vi "Test ModbusOverMOXA API.vi"() -> ()   [LabVIEW 2017]
doc: "ModbusOverMOXA API Tester."
uses:
  ModbusOverMOXA.lvlib
panel:
  in  "Write":bool
  in  "Read":bool
  in  "Len/Data":u16=1 format="%.0x"
  in  "Register":u16 format="%.0x"
  in  "Drive":bool
  in  "Hz":dbl
  in  "engage":bool
  in  "Boolean":bool
  in  "Status":bool
  in  "Local":bool
  in  "Remote":bool
  in  "config":string="{\"MQTT\":\"{\\n  \\\"Broker\\\": {\\n    \\\"IP\\\": \\\"192.168.20.249\\\",\\n    \\\"port\\\": 1883,\\n    \\\"connTimeout\\\": 3000,\\n    \\\"writeTimeout\\\": 3000,\\n    \\\"readTimeout\\\": 3000,\\n    \\\"subTimeout\\\": 3000\\n  },\\n  \\\"Connect Flags\\\": {\\n    \\\"reserved\\\": false,\\n    \\\"clean session\\\": false,\\n    \\\"will flag\\\": true,\\n    \\\"willQOS\\\": \\\"At least once\\\",\\n    \\\"will retain\\\": true,\\n    \\\"password\\\": false,\\n    \\\"user name\\\": false\\n  },\\n  \\\"Keep Alive\\\": 5000,\\n  \\\"Client Info\\\": {\\n    \\\"ClientId\\\": \\\"INVerterDriver$$$$$\\\",\\n    \\\"Will Topic\\\": \\\"InverterDriver/Online\\\",\\n    \\\"Will Message\\\": \\\"flase\\\",\\n    \\\"User Name\\\": \\\"\\\",\\n    \\\"Password\\\": \\\"\\\"\\n  }\\n}\",\"Serializer\":\"{\\n  \\\"Plugin\\\":\\\"MOXAIP\\\",\\n  \\\"IP\\\":\\\"192.168.20.119\\\",\\n  \\\"Port\\\":4002\\n}\",\"Messages\":\"{\\n  \\\"Subscriptions\\\":\\n  {\\n    \\\"Engage\\\":\\\"Inverter/Engage\\\",\\n    \\\"Drive\\\":\\\"Inverter/Drive\\\"\\n  },\\n  \\\"Broadcasts\\\":\\n  {\\n    \\\"Status\\\":\\\"Inverter/Status\\\"\\n  }\\n}\"}"
  in  "Settings Button":bool
  in  "Run as Singleton?":bool
  in  "Show Block Diagram":bool
  in  "Refresh Modules":bool
  out "Active Modules":string[](array[string])
  in  "Stop Module":bool
  in  "Select Module":i32(ring)=-1 caption="Select Module\nTo send Request to" items=["All"=-1]
  in  "Run New Module":bool
  in  "Hide Module Panel":bool
  in  "Show Module Panel":bool
  out "Status":string
  # "This VI tests the API for the Module."
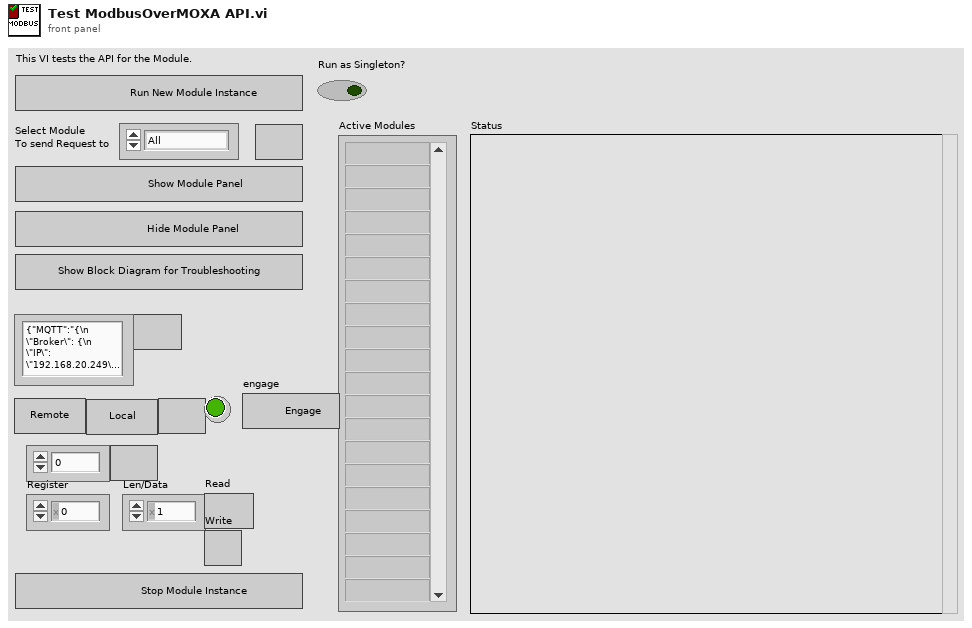
[diagram p1: front panel]
types:
  T1 = typedef "ModbusOverMOXA.lvlib/Broadcast Events--cluster.ctl" = cluster{"Module Did Init":refnum<user-event>, "Status Updated":refnum<user-event>, "Error Reported":refnum<user-event>, "Module Did Stop":refnum<user-event>, "Update Module Execution Status":refnum<user-event>}
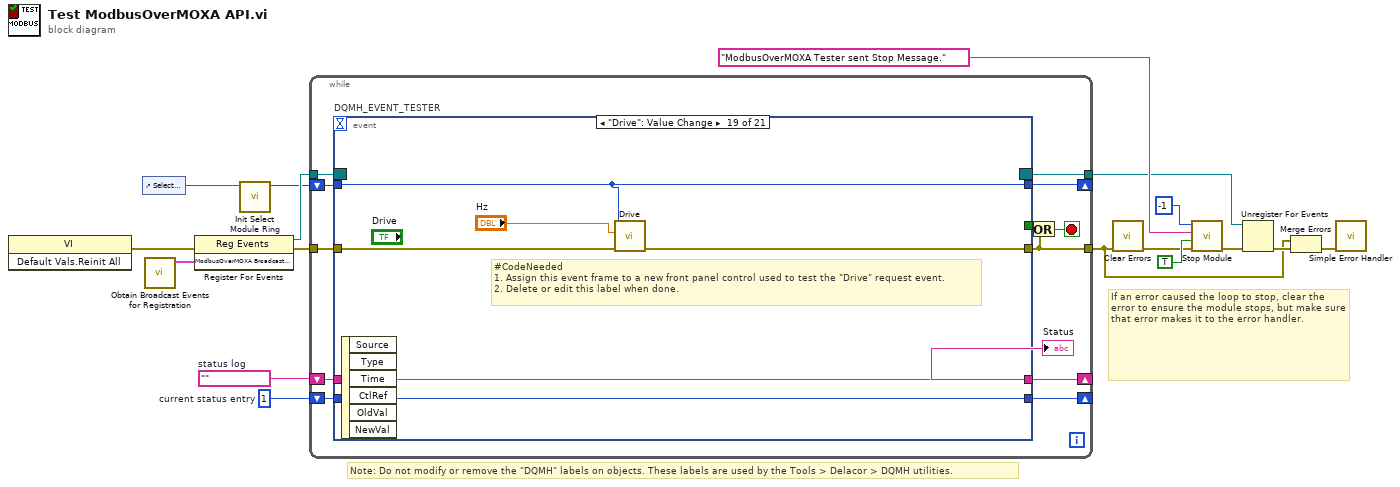
[diagram p0: block diagram]
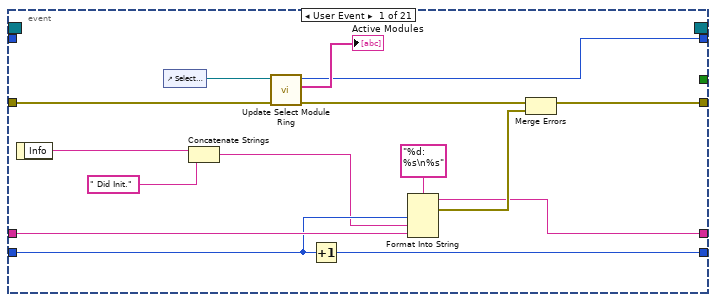
[diagram p2: hidden frame]
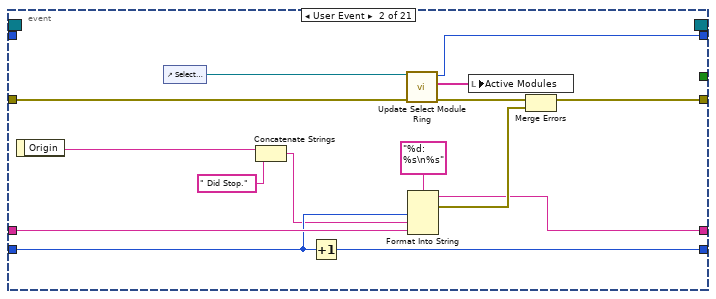
[diagram p3: hidden frame]
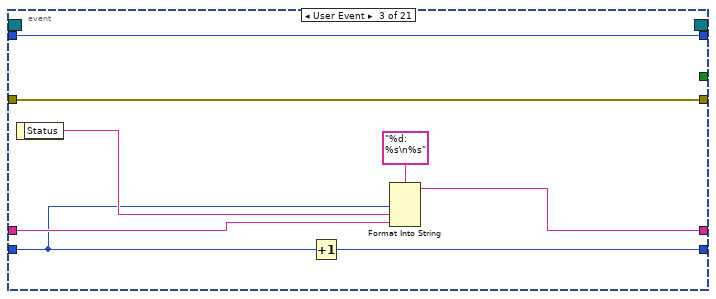
[diagram p4: hidden frame]
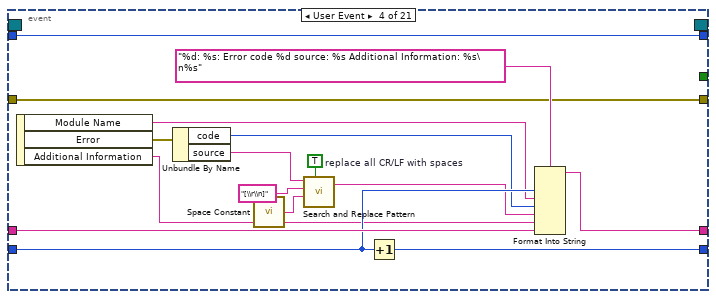
[diagram p5: hidden frame]
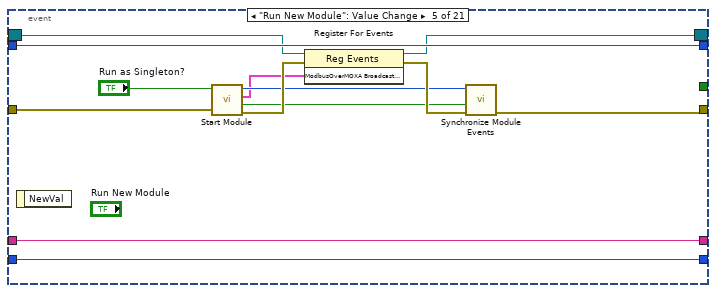
[diagram p6: hidden frame]
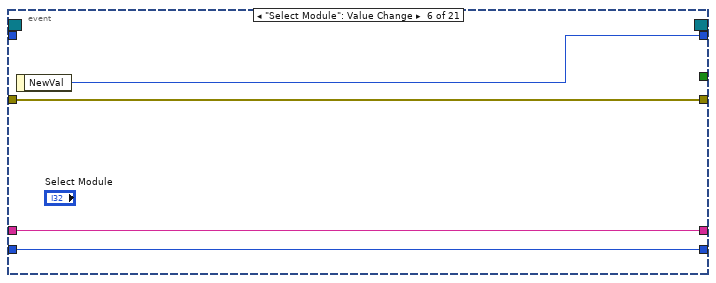
[diagram p7: hidden frame]
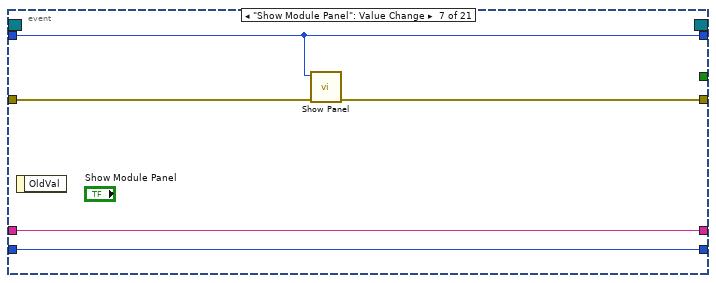
[diagram p8: hidden frame]
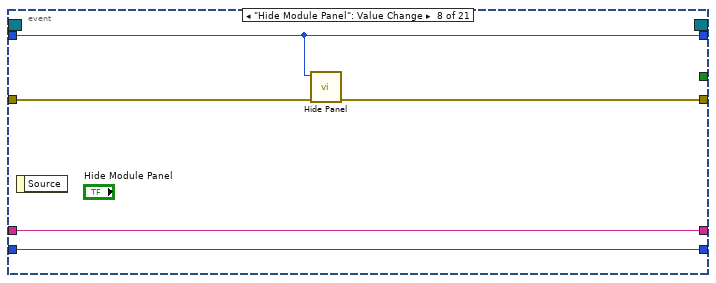
[diagram p9: hidden frame]
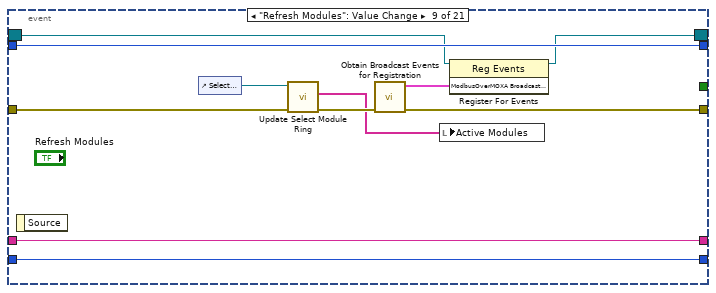
[diagram p10: hidden frame]
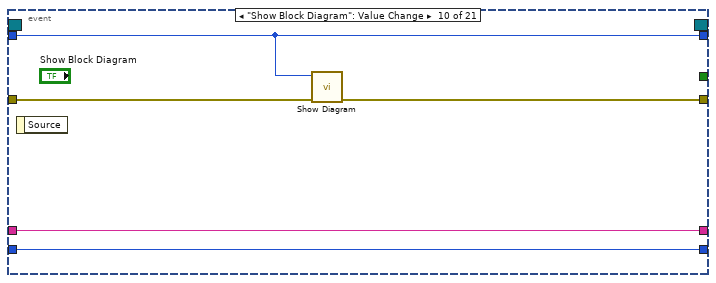
[diagram p11: hidden frame]
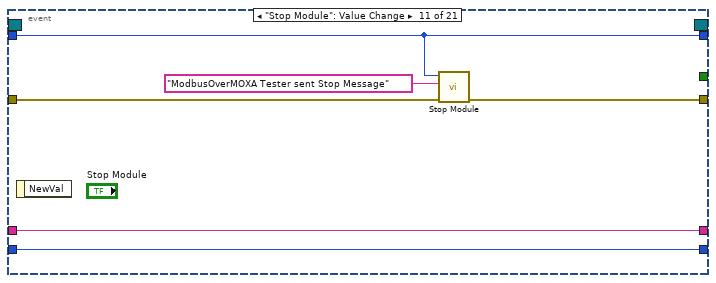
[diagram p12: hidden frame]
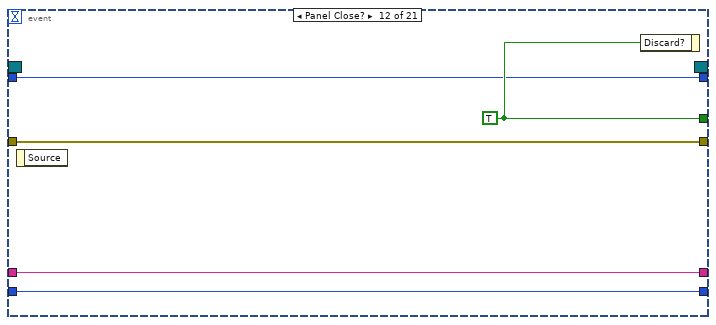
[diagram p13: hidden frame]
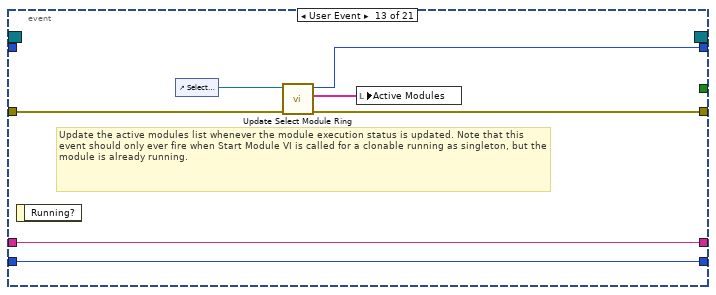
[diagram p14: hidden frame]
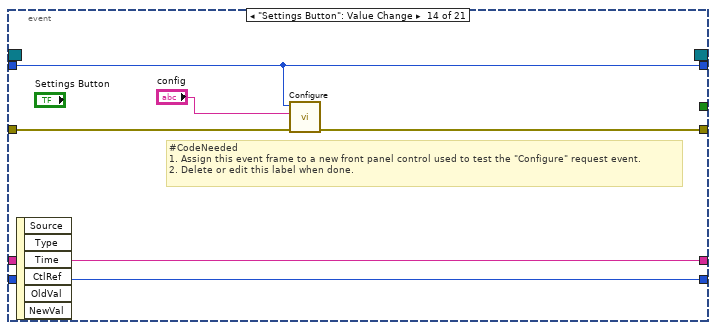
[diagram p15: hidden frame]
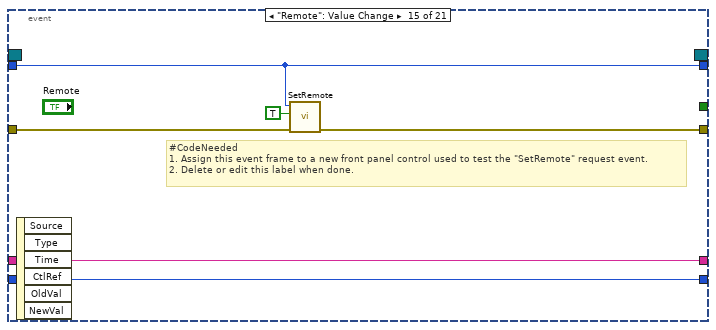
[diagram p16: hidden frame]
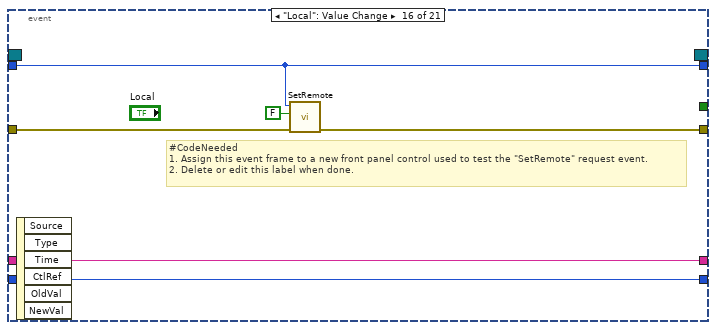
[diagram p17: hidden frame]
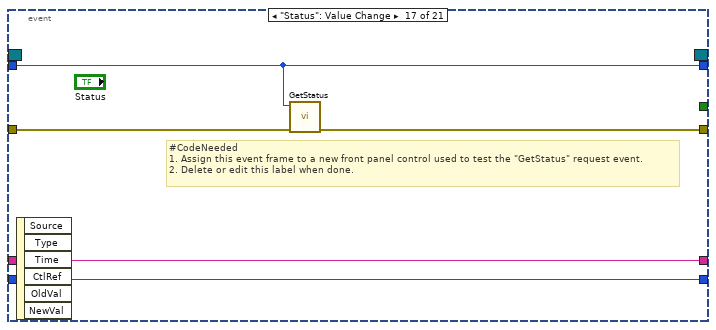
[diagram p18: hidden frame]
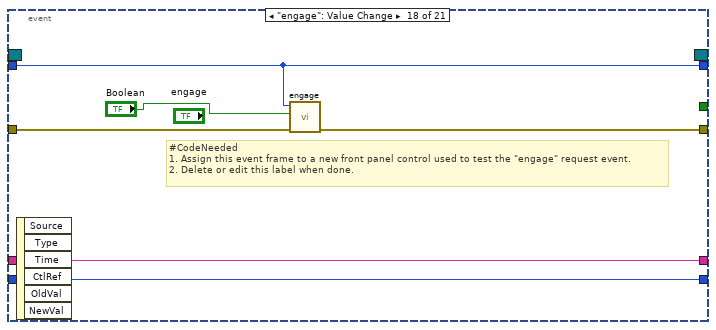
[diagram p19: hidden frame]
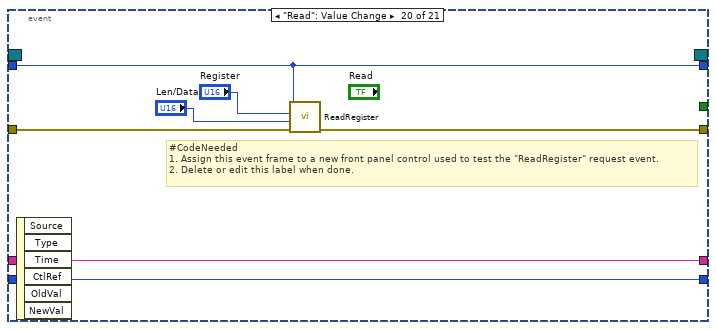
[diagram p20: hidden frame]
diagram:
  w13 = 1  # current status entry
  w14 = ""  # status log
  # "If an error caused the loop to stop, clear the error to ensure the module stops, but make sure that error makes it to the error handler."
  # "Note: Do not modify or remove the \"DQMH\" labels on objects. These labels are used by the Tools > Delacor > DQMH utilities."
  n1 = invoke class="VI" method="Default Vals.Reinit All"() -> (error out=w6:errorcluster)  [unwired: 3 in, 2 out]
  n2 = control-ref of="Select Module"() -> (w11:refnum<vi>)
  n3 = call "Obtain Broadcast Events for Registration.vi"() -> ("ModbusOverMOXA Broadcast Events"=w10:T1)  [unwired: 10 in, 1 out]
  n4 = register-events(error in=w6, w10) -> (reference out=w17:refnum<event-registration>, error out=w9:errorcluster)  [unwired: 1 in]
  n5 = call "Init Select Module Ring.vi"("Select Module Ring Ref"=w11) -> ("Value for All Modules"=w12:i32)  [unwired: 8 in, 2 out]
  n6 = while {
    tunnel: w17 -> [w29]
    tunnel: [w18] -> w1
    tunnel: w9 -> [w27]
    shift-right: [w23] -> _
    shift-left: w14 -> [w25]
    shift-right: [w24] -> _
    shift-left: w13 -> [w26]
    shift-right: [w20] -> _
    shift-left: w12 -> [w21]
    tunnel: [w19] -> w5
    stop <- w22 stop-if-true
    n7 = event "DQMH_EVENT_TESTER" shown="[18] \"Drive\": Value Change" {
      selector: w29 -> [_ _ _ _ w90 _ _ _ w116 _ _ _ _ _ _ _ _ _ _ _ _]
      dyn-events: [_ _ _ _ w89 _ _ _ w115 _ _ _ _ _ _ _ _ _ _ _ _] -> w19
      timeout: _ -> [_ _ _ _ _ _ _ _ _ _ _ _ _ _ _ _ _ _ _ _ _]
      tunnel: [_ _ _ _ _ _ _ _ _ _ _ w137 _ _ _ _ _ _ _ _ _] -> w28
      tunnel: [w33 w51 w67 w73 w88 w100 w104 w109 w112 w123 w128 w136 w140 w147 w153 w159 w164 w170 w176 w183 w190] -> w18
      tunnel: w27 -> [w35 w53 w67 w73 w91 w100 w105 w110 w117 w126 w129 w136 w141 w150 w156 w162 w167 w173 w179 w186 w193]
      tunnel: w26 -> [w41 w56 w60 w79 w93 w98 w102 w107 w120 w124 w131 w134 w143 w148 w154 w160 w165 w171 w177 w184 w191]
      tunnel: w25 -> [w42 w57 w63 w81 w94 w99 w103 w108 w121 w125 w132 w135 w144 w149 w155 w161 w166 w172 w178 w185 w192]
      tunnel: [w39 w54 w64 w76 w94 w99 w103 w108 w121 w125 w132 w135 w144 w149 w155 w161 w166 w172 w178 w185 w192] -> w23
      tunnel: [w40 w55 w66 w82 w93 w98 w102 w107 w120 w124 w131 w134 w143 w148 w154 w160 w165 w171 w177 w184 w191] -> w24
      tunnel: w21 -> [_ _ w61 w83 w92 _ w101 w106 w119 w122 w130 w133 _ w145 w152 w158 w163 w169 w174 w181 w189]
      tunnel: [w30 w48 w61 w83 w92 w97 w101 w106 w119 w122 w130 w133 w139 w145 w152 w158 w163 w169 w174 w181 w189] -> w20
      event User Event {
        n8 = event-data() -> ("Info"=w38:string)  [unwired: 1 in]
        n9 = control-ref of="Select Module"() -> (w32:refnum<vi>)
        n10 = Concatenate Strings(w38, " Did Init.") -> (w37:string)
        n11 = call "Update Select Module Ring.vi"("error in (no error)"=w35, "Select Module Ring Ref"=w32) -> ("error out"=w34:errorcluster, "Active Modules (Array)"=→"Active Modules":string[], "New Module Ring Value"=w30:i32)  [unwired: 7 in]
        n12 = Increment(x=w41) -> (x+1=w40:i32)
        n13 = Format Into String(format string="%d: %s\n%s", w41, w37, w42) -> (resulting string=w39:string, error out=w44:errorcluster)  [unwired: 2 in]
        n14 = Merge Errors(w34, w44) -> (w33:errorcluster)
      }
      event User Event {
        n15 = event-data() -> ("Origin"=w46:string)  [unwired: 1 in]
        n16 = control-ref of="Select Module"() -> (w50:refnum<vi>)
        n17 = Concatenate Strings(w46, " Did Stop.") -> (w45:string)
        n18 = Increment(x=w56) -> (x+1=w55:i32)
        n19 = call "Update Select Module Ring.vi"("error in (no error)"=w53, "Select Module Ring Ref"=w50) -> ("error out"=w52:errorcluster, "Active Modules (Array)"=w49:string[], "New Module Ring Value"=w48:i32)  [unwired: 7 in]
        n20 = Format Into String(format string="%d: %s\n%s", w56, w45, w57) -> (resulting string=w54:string, error out=w59:errorcluster)  [unwired: 2 in]
        n21 = local write "Active Modules"(w49) -> ()
        n22 = Merge Errors(w52, w59) -> (w51:errorcluster)
      }
      event User Event {
        n23 = event-data() -> ("Status"=w62:string)  [unwired: 1 in]
        n24 = Increment(x=w60) -> (x+1=w66:i32)
        n25 = Format Into String(format string="%d: %s\n%s", w60, w62, w63) -> (resulting string=w64:string)  [unwired: 2 in, 1 out]
      }
      event User Event {
        w77 = TRUE  # replace all CR/LF with spaces
        n26 = event-data() -> ("Module Name"=w71:string, "Error"=w70:errorcluster, "Additional Information"=w68:string)  [unwired: 1 in]
        n27 = Unbundle By Name(w70) -> ("code"=w72:i32, "source"=w74:string)
        n28 = call <vilib>:"Space Constant.vi"() -> ("String"=w78:string)
        n29 = call <vilib>:"Search and Replace Pattern.vi"("string"=w74, "regular expression (\"\")"="[\\r\\n]" ("regular expression (\"\")"), "replace string (\"\")"=w78, "replace all? (F)"=w77) -> ("result string"=w75:string)  [unwired: 1 in, 1 out]
        n30 = Increment(x=w79) -> (x+1=w82:i32)
        n31 = Format Into String(format string="%d: %s: Error code %d source: %s Additional Information: %s\n%s", w79, w71, w72, w75, w68, w81) -> (resulting string=w76:string)  [unwired: 2 in, 1 out]
      }
      event "Run New Module": Value Change {
        n32 = event-data() -> ()  [unwired: 1 in, 1 out]
        n33 = call "Start Module.vi"("error in (no error)"=w91, "Run as Singleton? (F)"="Run as Singleton?") -> ("error out"=w95:errorcluster, "Wait for Event Sync?"=w86:bool, "ModbusOverMOXA Broadcast Events"=w85:T1, "Module ID"=w87:i32)  [unwired: 6 in]
        n34 = register-events(reference=w90, error in=w95, w85) -> (reference out=w89:refnum<event-registration>, error out=w96:errorcluster)
        n35 = call "Synchronize Module Events.vi"("error in (no error)"=w96, "Wait for Event Sync?"=w86, "Module ID"=w87) -> ("error out"=w88:errorcluster)  [unwired: 7 in, 1 out]
      }
      event "Select Module": Value Change {
        n36 = event-data() -> ("NewVal"=w97:i32)  [unwired: 1 in]
      }
      event "Show Module Panel": Value Change {
        n37 = event-data() -> ()  [unwired: 1 in, 1 out]
        n38 = call "Show Panel.vi"("error in (no error)"=w105, "Module ID"=w101) -> ("error out"=w104:errorcluster)  [unwired: 9 in]
      }
      event "Hide Module Panel": Value Change {
        n39 = event-data() -> ()  [unwired: 1 in, 1 out]
        n40 = call "Hide Panel.vi"("error in (no error)"=w110, "Module ID"=w106) -> ("error out"=w109:errorcluster)  [unwired: 9 in]
      }
      event "Refresh Modules": Value Change {
        n41 = event-data() -> ()  [unwired: 1 in, 1 out]
        n42 = control-ref of="Select Module"() -> (w118:refnum<vi>)
        n43 = call "Update Select Module Ring.vi"("error in (no error)"=w117, "Select Module Ring Ref"=w118) -> ("error out"=w113:errorcluster, "Active Modules (Array)"=w111:string[])  [unwired: 7 in, 1 out]
        n44 = call "Obtain Broadcast Events for Registration.vi"("error in (no error)"=w113) -> ("error out"=w112:errorcluster, "ModbusOverMOXA Broadcast Events"=w114:T1)  [unwired: 9 in]
        n45 = local write "Active Modules"(w111) -> ()
        n46 = register-events(reference=w116, w114) -> (reference out=w115:refnum<event-registration>)  [unwired: 1 in, 1 out]
      }
      event "Show Block Diagram": Value Change {
        n47 = event-data() -> ()  [unwired: 1 in, 1 out]
        n48 = call "Show Diagram.vi"("error in (no error)"=w126, "Module ID"=w122) -> ("error out"=w123:errorcluster)  [unwired: 9 in]
      }
      event "Stop Module": Value Change {
        n49 = event-data() -> ()  [unwired: 1 in, 1 out]
        n50 = call "Stop Module.vi"("error in (no error)"=w129, "Origin"="ModbusOverMOXA Tester sent Stop Message", "Module ID"=w130) -> ("error out"=w128:errorcluster)  [unwired: 8 in]
      }
      event Panel Close? {
        w137 = TRUE ("Discard?")
        n51 = event-data() -> ()  [unwired: 1 in, 1 out]
        n52 = event-data("Discard?"=w137) -> ()  [unwired: 1 in, 1 out]
      }
      event User Event {
        # "Update the active modules list whenever the module execution status is updated. Note that this event should only ever fire when Start Module VI is called for a clonable running as singleton, but the module is already running."
        n53 = event-data() -> ()  [unwired: 1 in, 1 out]
        n54 = control-ref of="Select Module"() -> (w142:refnum<vi>)
        n55 = call "Update Select Module Ring.vi"("error in (no error)"=w141, "Select Module Ring Ref"=w142) -> ("error out"=w140:errorcluster, "Active Modules (Array)"=w138:string[], "New Module Ring Value"=w139:i32)  [unwired: 7 in]
        n56 = local write "Active Modules"(w138) -> ()
      }
      event "Settings Button": Value Change {
        # "#CodeNeeded\n1. Assign this event frame to a new front panel control used to test the \"Configure\" request event.\n2. Delete or edit this label when done."
        n57 = event-data() -> ()  [unwired: 1 in, 6 out]
        n58 = call "Configure.vi"("error in (no error)"=w150, "Jsonconfig"="config", "Module ID"=w145) -> ("error out"=w147:errorcluster)  [unwired: 8 in]
      }
      event "Remote": Value Change {
        # "#CodeNeeded\n1. Assign this event frame to a new front panel control used to test the \"SetRemote\" request event.\n2. Delete or edit this label when done."
        n59 = event-data() -> ()  [unwired: 1 in, 6 out]
        n60 = call "SetRemote.vi"("error in (no error)"=w156, "Remote?"=TRUE, "Module ID"=w152) -> ("error out"=w153:errorcluster)  [unwired: 8 in]
      }
      event "Local": Value Change {
        # "#CodeNeeded\n1. Assign this event frame to a new front panel control used to test the \"SetRemote\" request event.\n2. Delete or edit this label when done."
        n61 = event-data() -> ()  [unwired: 1 in, 6 out]
        n62 = call "SetRemote.vi"("error in (no error)"=w162, "Remote?"=FALSE, "Module ID"=w158) -> ("error out"=w159:errorcluster)  [unwired: 8 in]
      }
      event "Status": Value Change {
        # "#CodeNeeded\n1. Assign this event frame to a new front panel control used to test the \"GetStatus\" request event.\n2. Delete or edit this label when done."
        n63 = event-data() -> ()  [unwired: 1 in, 6 out]
        n64 = call "GetStatus.vi"("error in (no error)"=w167, "Module ID"=w163) -> ("error out"=w164:errorcluster)  [unwired: 9 in]
      }
      event "engage": Value Change {
        # "#CodeNeeded\n1. Assign this event frame to a new front panel control used to test the \"engage\" request event.\n2. Delete or edit this label when done."
        n65 = event-data() -> ()  [unwired: 1 in, 6 out]
        n66 = call "engage.vi"("error in (no error)"=w173, "Engage"="Boolean", "Module ID"=w169) -> ("error out"=w170:errorcluster)  [unwired: 8 in]
      }
      event "Drive": Value Change {
        # "#CodeNeeded\n1. Assign this event frame to a new front panel control used to test the \"Drive\" request event.\n2. Delete or edit this label when done."
        n67 = event-data() -> ()  [unwired: 1 in, 6 out]
        n68 = call "Drive.vi"("error in (no error)"=w179, "Hz"="Hz", "Module ID"=w174) -> ("error out"=w176:errorcluster)  [unwired: 8 in]
      }
      event "Read": Value Change {
        # "#CodeNeeded\n1. Assign this event frame to a new front panel control used to test the \"ReadRegister\" request event.\n2. Delete or edit this label when done."
        n69 = event-data() -> ()  [unwired: 1 in, 6 out]
        n70 = call "ReadRegister.vi"("error in (no error)"=w186, "Length"="Len/Data", "Register"="Register", "Module ID"=w181) -> ("error out"=w183:errorcluster)  [unwired: 7 in]
      }
      event "Write": Value Change {
        # "#CodeNeeded\n1. Assign this event frame to a new front panel control used to test the \"WriteRegister\" request event.\n2. Delete or edit this label when done."
        n71 = event-data() -> ()  [unwired: 1 in, 6 out]
        n72 = local read "Register"() -> (w188:u16)
        n73 = local read "Len/Data"() -> (w187:u16)
        n74 = call "WriteRegister.vi"("error in (no error)"=w193, "Data"=w187, "Register"=w188, "Module ID"=w189) -> ("error out"=w190:errorcluster)  [unwired: 7 in]
      }
    }
    "Status" <- w23
    n75 = Or(x=w28, y=w18) -> (x .or. y?=w22:bool)
  }
  n76 = call <vilib>:"Clear Errors.vi"("error in (no error)"=w1) -> ("error out"=w3:errorcluster)  [unwired: 5 in, 1 out]
  n77 = call "Stop Module.vi"("error in (no error)"=w3, "Wait for Module to stop? (F)"=TRUE ("Wait for Module to stop?"), "Origin"="ModbusOverMOXA Tester sent Stop Message.", "Module ID"=-1 ("Stop all")) -> ("error out"=w15:errorcluster)  [unwired: 7 in]
  n78 = Unregister For Events(event registration refnum=w5, error in=w15) -> (error out=w16:errorcluster)
  n79 = Merge Errors(w1, w16) -> (w2:errorcluster)
  n80 = call <vilib>:"Simple Error Handler.vi"("error in (no error)"=w2) -> ()  [unwired: 4 in, 5 out]
